vi "adipiezomeasure20242.vi"() -> ()   [LabVIEW 2020]
uses:
  <vilib>/Analysis/NI_AALPro.lvlib
  <vilib>/Analysis/2dsp.llb/Real FFT.vi
panel:
  out "Save to:":path caption="File Name Out"
  out "Saving":bool
  in  "Record":bool
  in  "Sample Name":string(combo)="4200g"
  in  "rate":dbl=40000.0
  in  "number of samples":i32=4000
  out "Spectrum":dynamicdata(graph) caption="data"
  out "Piezos":dynamicdata(graph) caption="data"
  in  "stop 2":bool
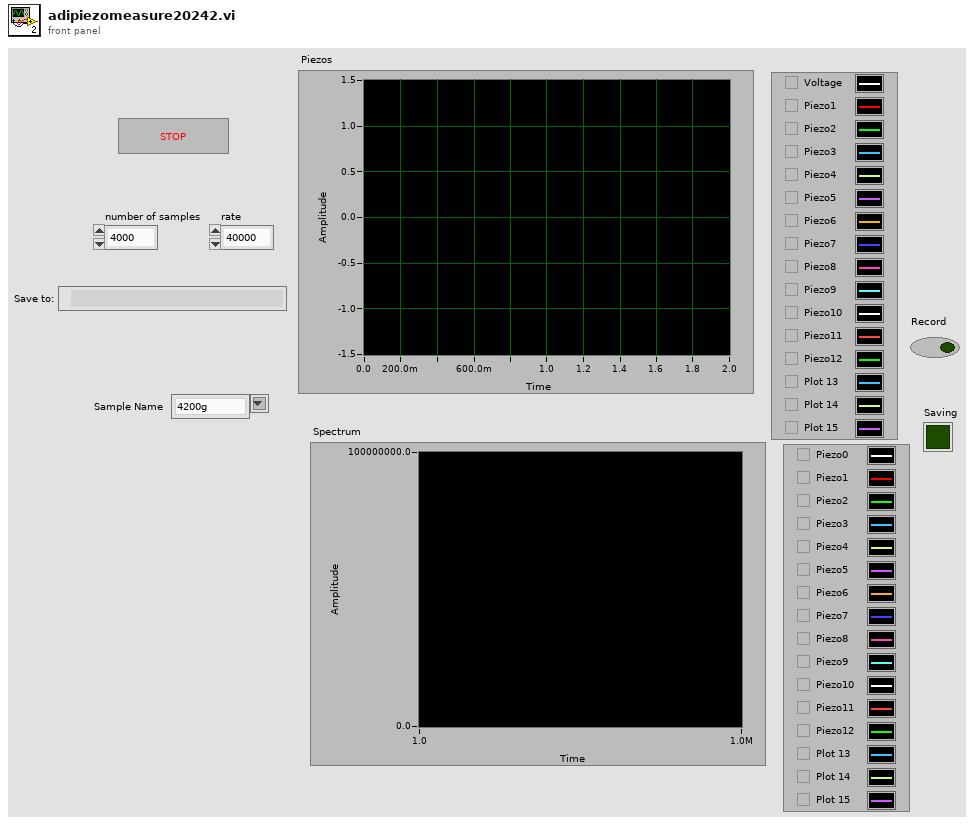
[diagram p1: front panel]
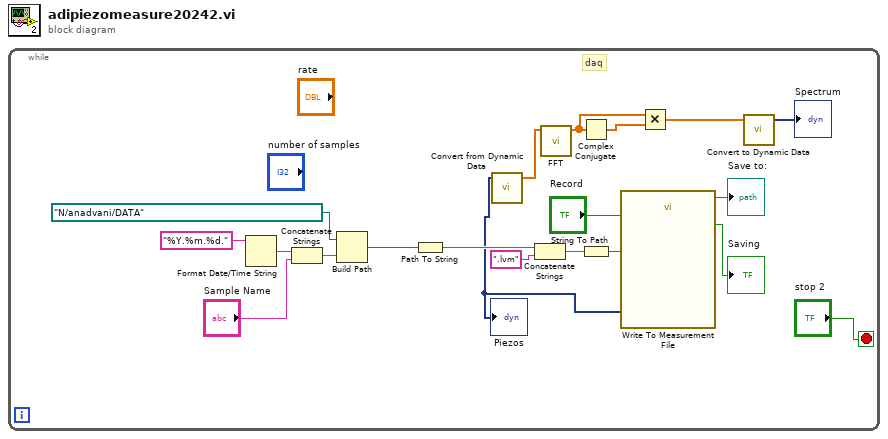
[diagram p0: block diagram]
diagram:
  n1 = while {
    stop <- "stop 2" stop-if-true
    # "daq"
    n2 = Format Date/Time String(time format string (%c)="%Y.%m.%d.") -> (date/time string=w13:string)  [unwired: 2 in]
    n3 = Concatenate Strings(w13, "Sample Name") -> (w14:string)
    n4 = Build Path(base path=path "N:/anadvani/DATA", name or relative path=w14) -> (appended path=w4:path)
    n5 = Path To String(path=w4) -> (string=w12:string)
    n6 = call "Convert from Dynamic Data"("Dynamic Data Type"="Piezos") -> ("Array"=w19:dbl[])  [unwired: 3 in]
    n7 = Concatenate Strings(w12, ".lvm" ("string")) -> (w10:string)
    n8 = call-poly <vilib>:"FFT.vi"("X"=w19) -> ("FFT {X}"=w21:cdb[])  [unwired: 9 in, 1 out]
    n9 = Complex Conjugate(1:w21) -> (0:w20:cdb[])
    n10 = String To Path(string=w10) -> (path=w9:path)
    n11 = call "Write To Measurement File"("Signals"="Piezos", "Enable"="Record", "Filename"=w9) -> ("Filename Out"=→"Save to:":path, "Saving Data"=→"Saving":bool)  [unwired: 14 in, 1 out]
    n12 = Multiply(x=w21, y=w20) -> (x*y=w18:cdb[])
    n13 = call "Convert to Dynamic Data"("Array"=w18) -> ("Dynamic Data Type"=→"Spectrum":dynamicdata)  [unwired: 3 in]
  }
